vi "measure_i.vi"(8 "error in (no error)":errorcluster, 10 "Channel":string="1", 11 "VISA Refnum in":refnum<visa-resource-name>) -> (0 "error out":errorcluster, 2 "I readback (A)":dbl, 3 "VISA Refnum out":refnum<visa-resource-name>)   [LabVIEW 2018, in "Aim-TTi CPX400SP.lvlib"]
uses:
  <instrlib>/Aim-TTi CPX400SP/Aim-TTi CPX400SP.lvlib
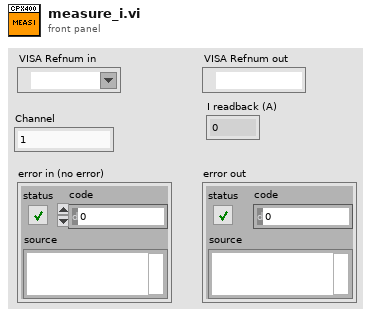
[diagram p1: front panel]
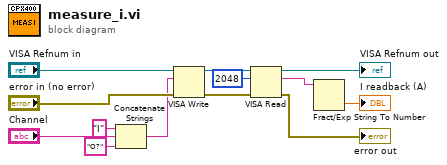
[diagram p0: block diagram]
diagram:
  n1 = Concatenate Strings("I" ("string"), "Channel", "O?" ("string")) -> (w3:string)
  n2 = VISA Write(VISA resource name="VISA Refnum in", write buffer=w3, error in (no error)="error in (no error)") -> (VISA resource name out=w7:refnum<visa-resource-name>, error out=w8:errorcluster)  [unwired: 1 out]
  n3 = VISA Read(VISA resource name=w7, byte count=u32 2048, error in (no error)=w8) -> (VISA resource name out=→"VISA Refnum out":refnum<visa-resource-name>, read buffer=w2:string, error out=→"error out":errorcluster)  [unwired: 1 out]
  n4 = Fract/Exp String To Number(string=w2) -> (number=→"I readback (A)":dbl)  [unwired: 3 in, 1 out]
